vi "CloseDotNetReferenceInClusterArray.vi"(1 "Array Of .NET Refs":cluster{".NET Refnum":refnum<k24>}[](array[cluster])) -> (0 "error out":errorcluster)   [LabVIEW 2010]
uses:
  \\camila\f$/Tests/LVBuildValidation/10.0/Automated/FlexLVAdapter30/Refnums/DotNetRefnum/LabviewDNTest.dll
  LabviewDNTest.dll
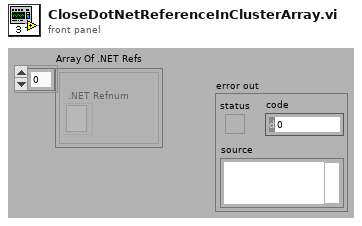
[diagram p1: front panel]
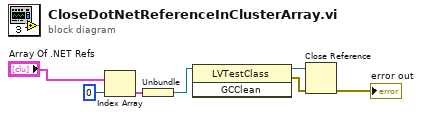
[diagram p0: block diagram]
diagram:
  n1 = Index Array(array="Array Of .NET Refs", index=0) -> (element=w4:cluster{".NET Refnum":refnum<k24>})
  n2 = Unbundle(w4) -> (".NET Refnum"=w1:refnum<k24>)
  n3 = invoke class="LVTestClass" method="GCClean"(reference=w1) -> (reference out=w2:refnum<k24>, error out=w3:errorcluster)  [unwired: 2 in, 1 out]
  n4 = Close Reference(reference=w2, error in (no error)=w3) -> (error out=→"error out":errorcluster)
